vi "toml_is_loaded.vi"(4 "vi":refnum<vi>, 8 "error in (no error)":errorcluster, 11 "path in":path) -> (0 "error out":errorcluster, 1 "toml":string, 2 "file loaded":bool, 3 "path out":path)   [LabVIEW 2017]
uses:
  <vilib>/Utility/error.llb/Clear Errors.vi
  toml_lock_obtain.vi
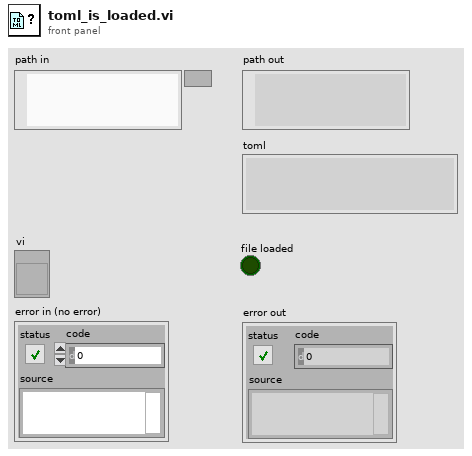
[diagram p1: front panel]
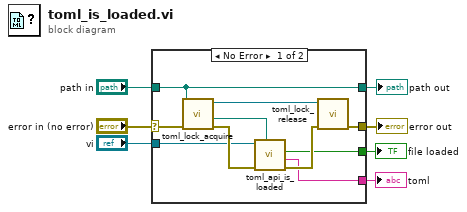
[diagram p0: block diagram]
diagram:
  n1 = case shown="No Error" "error in (no error)" {
    selector: "error in (no error)" -> [w16 w18]
    tunnel: [w15 w18] -> w6
    tunnel: "vi" -> [w12 _]
    tunnel: "path in" -> [w14 w19]
    tunnel: [w14 w19] -> w3
    tunnel: [w9 _] -> w2
    tunnel: [w10 _] -> w1
    frame No Error {
      n2 = call "toml_lock_acquire.vi"("error in (no error)"=w16, "path in"=w14) -> ("error out"=w13:errorcluster, "resolved path"=w8:path, "lock"=w17:refnum<queue>)  [unwired: 7 in]
      n3 = call "toml_api_is_loaded.vi"("resolved path"=w8, "error in (no error)"=w13, "vi in"=w12) -> ("error out"=w11:errorcluster, "text"=w10:string, "file loaded"=w9:bool)  [unwired: 5 in, 1 out]
      n4 = call "toml_lock_release.vi"("error in (no error)"=w11, "lock"=w17) -> ("error out"=w15:errorcluster)  [unwired: 9 in]
    }
    frame Error {
    }
  }
  "error out" <- w6
  "path out" <- w3
  "file loaded" <- w2
  "toml" <- w1
